vi "gpib_ascii_terminal.vi"() -> ()   [LabVIEW 2013]
uses:
  <vilib>/Instr/_visa.llb/GPIB Status Boolean Array.ctl
panel:
  out "Read Status":T1
  out "data 2":string
  in  "byte count":i32
  out "Write Status":T1
  in  "data":string
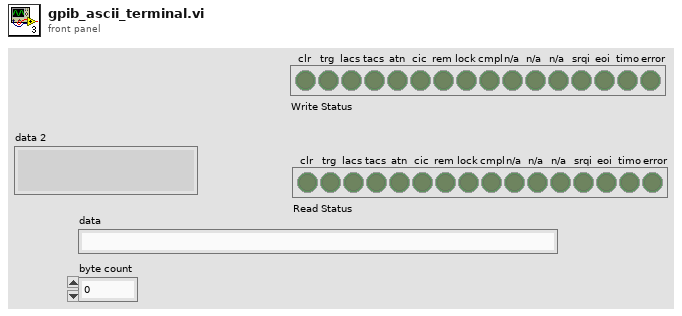
[diagram p1: front panel]
types:
  T1 = typedef "GPIB Status Boolean Array.ctl" = bool[]
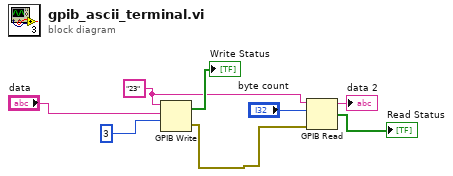
[diagram p0: block diagram]
diagram:
  w2 = "23" ("address string")
  n1 = GPIB Write(0:w2, 1:"data", 2:i16 3 ("mode (0)")) -> (5:→"Write Status":bool[], 6:w1:errorcluster)  [unwired: 2 in]
  n2 = GPIB Read(0:w2, 1:"byte count", 3:w1) -> (5:→"data 2":string, 6:→"Read Status":bool[])  [unwired: 2 in, 1 out]
